vi "CreateFeatureList.vi"(9 "feature display names":string[](array[string]), 10 "feature code names":string[](array[string])) -> (3 "feature lists":string[](array[string]))   [LabVIEW 2017, in "Tdms.lvlib"]
uses:
  <vilib>/addons/InsightCM/Utilities/Tdms/Tdms.lvlib
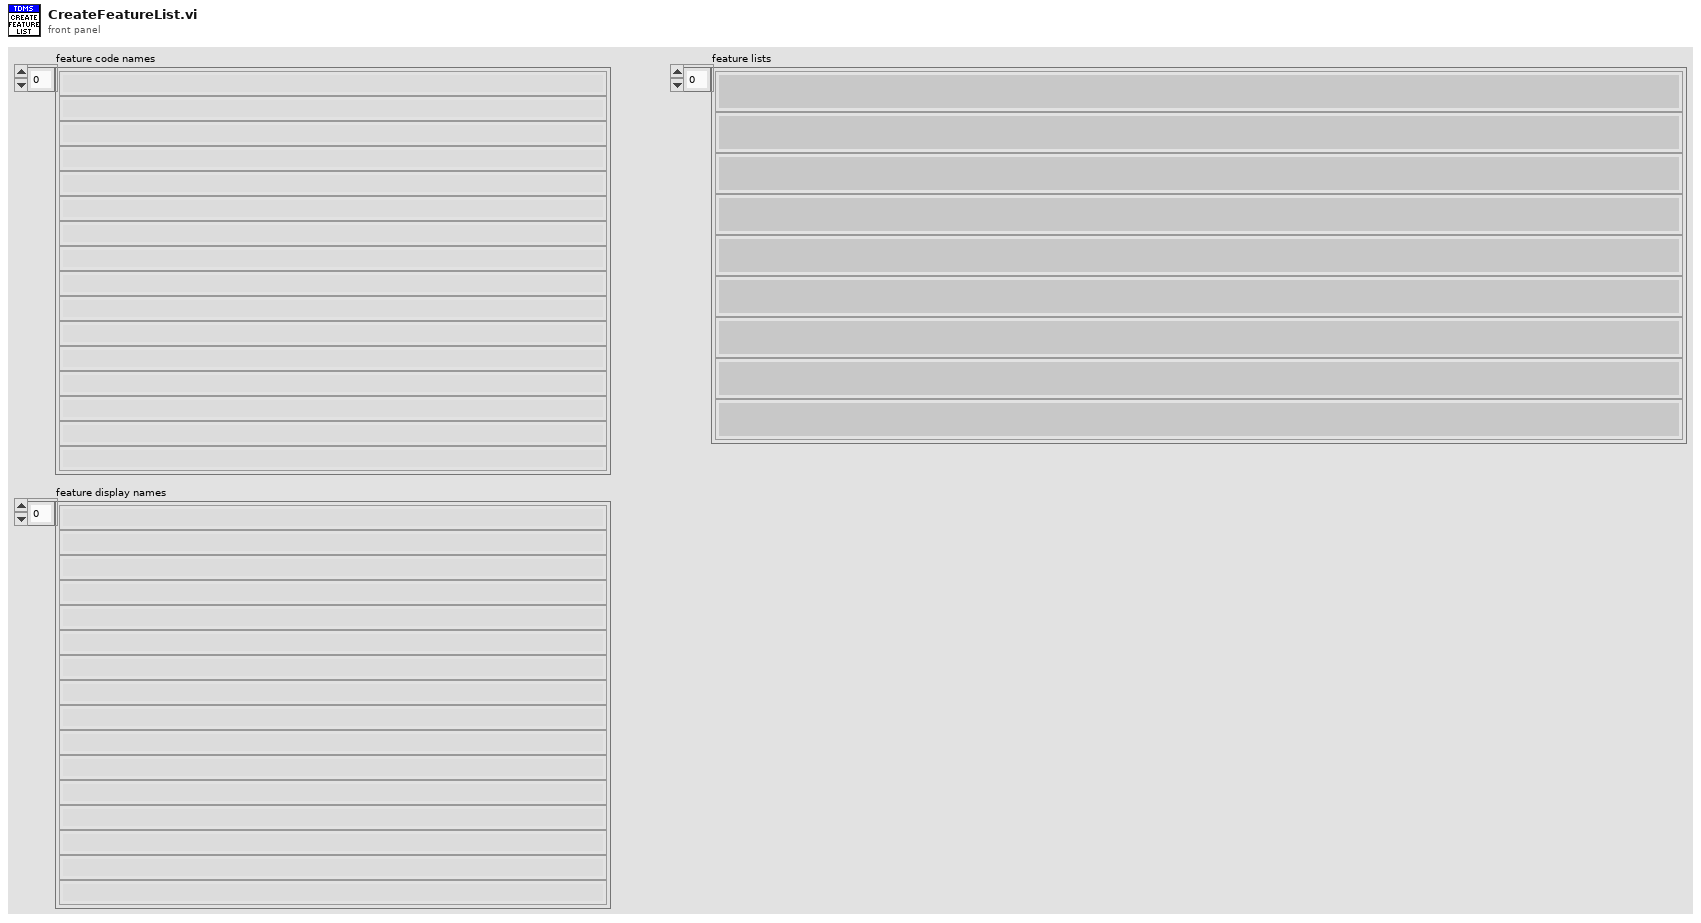
[diagram p1: front panel]
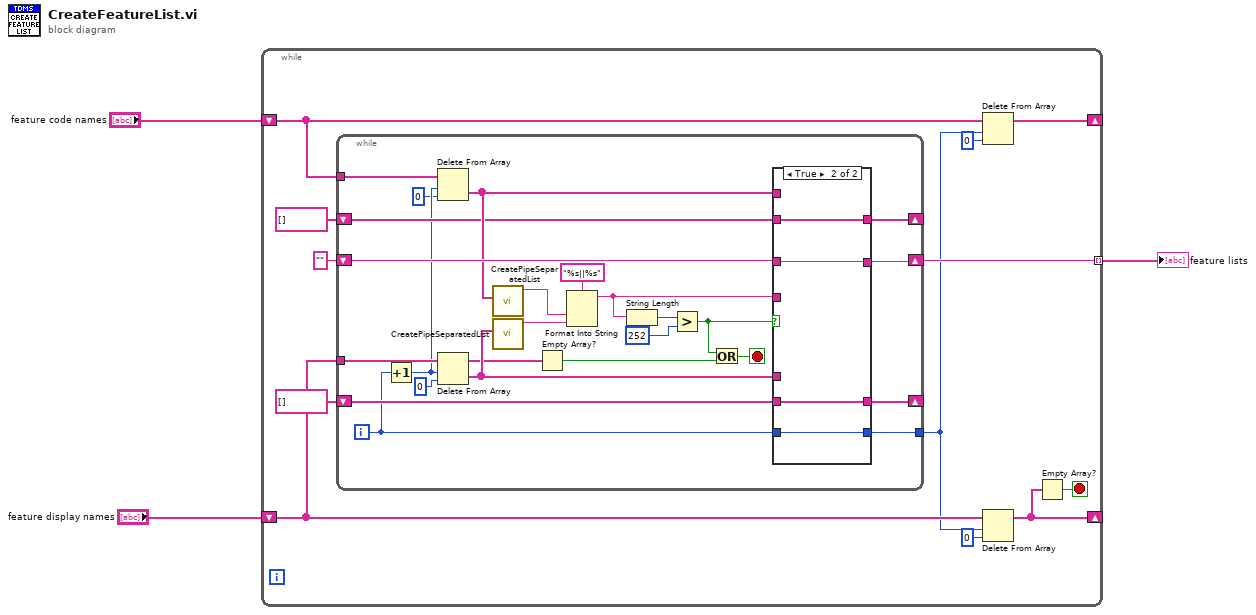
[diagram p0: block diagram]
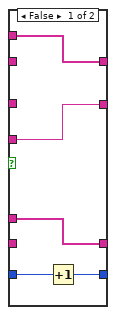
[diagram p2: hidden frame]
diagram:
  n1 = while {
    shift-right: [w10] -> _
    shift-left: "feature code names" -> [w11]
    shift-right: [w7] -> _
    shift-left: "feature display names" -> [w9]
    tunnel: [w12] -> w2 mode=indexing
    stop <- w6 stop-if-true
    n2 = while {
      tunnel: w11 -> [w35]
      tunnel: w9 -> [w28]
      shift-right: [w34] -> w12
      shift-left: "" -> [w32]
      shift-right: [w31] -> _
      shift-left: string[] [] ("Feature Code Names") -> [w29]
      shift-right: [w26] -> _
      shift-left: string[] [] ("Feature Display Names") -> [w25]
      tunnel: [w18] -> w8
      i -> [w17]
      stop <- w21 stop-if-true
      n3 = Increment(x=w17) -> (x+1=w20:i32)
      n4 = Delete From Array(array=w35, length=w20, index=0) -> (deleted portion=w30:string[])  [unwired: 1 out]
      n5 = Delete From Array(array=w28, length=w20, index=0) -> (deleted portion=w27:string[], array with subset deleted=w24:string[])
      n6 = call <vilib>:"CreatePipeSeparatedList.vi"("Array"=w30) -> ("List Out"=w39:string)  [unwired: 10 in]
      n7 = call <vilib>:"CreatePipeSeparatedList.vi"("Array"=w27) -> ("List Out"=w38:string)  [unwired: 10 in]
      n8 = Empty Array?(array=w24) -> (empty?=w22:bool)
      n9 = Format Into String(format string="%s||%s", w39, w38) -> (resulting string=w33:string)  [unwired: 2 in, 1 out]
      n10 = String Length(string=w33) -> (length=w37:i32)
      n11 = Greater?(x=w37, y=252) -> (0:w23:bool)
      n12 = Or(x=w23, y=w22) -> (x .or. y?=w21:bool)
      n13 = case shown="True" w23 {
        tunnel: [w45 w49] -> w34
        tunnel: w33 -> [w45 _]
        tunnel: w32 -> [_ w49]
        tunnel: [w44 w48] -> w31
        tunnel: w30 -> [w44 _]
        tunnel: w29 -> [_ w48]
        tunnel: w27 -> [w43 _]
        tunnel: [w43 w47] -> w26
        tunnel: w25 -> [_ w47]
        tunnel: [w41 w46] -> w18
        tunnel: w17 -> [w42 w46]
        frame False {
          n14 = Increment(x=w42) -> (x+1=w41:i32)
        }
        frame True {
        }
      }
    }
    n15 = Delete From Array(array=w11, length=w8, index=0) -> (array with subset deleted=w10:string[])  [unwired: 1 out]
    n16 = Delete From Array(array=w9, length=w8, index=0) -> (array with subset deleted=w7:string[])  [unwired: 1 out]
    n17 = Empty Array?(array=w7) -> (empty?=w6:bool)
  }
  "feature lists" <- w2
